vi "Boolean Text Write 2.vi"(4 "error in (no error)":errorcluster, 5 "Value":string, 6 "Container State":T2, 7 "Display State In":T1) -> (0 "error out":errorcluster, 3 "Display State Out":T1)   [LabVIEW 2019]
uses:
  <vilib>/_xctls/Container State.ctl
  System Button/State 1.ctl
  <vilib>/_xctls/XControlSupport.lvlib
  System Button/System Button.xctl
panel:
  # "Replace the Value Control below with a Control of desired type.\nDo not remove this Control or the others from the connector pane.\nDo not change the connector pane pattern.\nThe Value control should always be the third terminal from top on the input side in the connector pane."
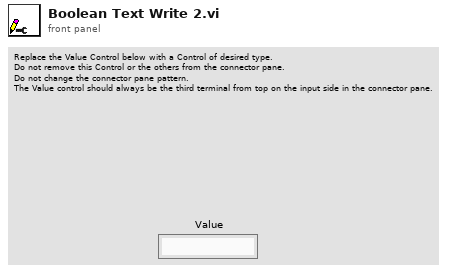
[diagram p1: front panel]
types:
  T1 = typedef "System Button.xctl/State 1.ctl" = cluster{"Armed":bool, "Acquiring":bool, "System Type":string, "System ID":string, "System ID Big":string}
  T2 = typedef "XControlSupport.lvlib/Container State.ctl" = cluster{"Indicator?":bool, "Run Mode?":bool, " Refnum":refnum<vi>}
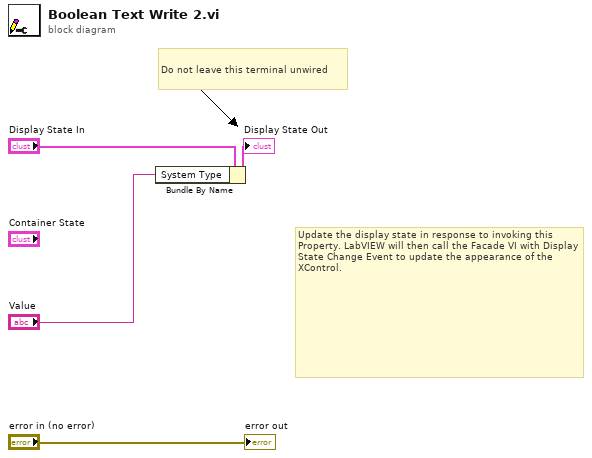
[diagram p0: block diagram]
diagram:
  # "Do not leave this terminal unwired"
  # "Update the display state in response to invoking this Property. LabVIEW will then call the Facade VI with Display State Change Event to update the appearance of the XControl."
  n1 = Bundle By Name(cluster="Display State In", "System Type"="Value") -> (→"Display State Out":T1)
  "error out" <- "error in (no error)"
